vi "Device.Init.vi"(8 "error in (no error)":errorcluster, 11 "OPM.ThorlabsPM400":refnum<class "OPM.ThorlabsPM400.lvclass">) -> (0 "error out":errorcluster, 2 "Result":bool, 3 "OPM.ThorlabsPM400 out":refnum<class "OPM.ThorlabsPM400.lvclass">)   [LabVIEW 2017, in "OPM.ThorlabsPM400.lvclass"]
doc: "---------------------------------------------------------------\nJKI State Machine Objects™\nhttp://jki.net/state-machine-objects/\nCopyright (C) 2005-2015, JKI <info@jki.net>\nALL RIGHTS RESERVEDJKI State Machine Objects (SMO) 1.0.0.5\nJKI - JKI\nCopyright (c) 2016, JKI"
uses:
  OPM.ThorlabsPM400.lvclass
  D:/upwork/Laser Measurement Tool/Laser/project/Subsystems/OPM/OPM.lvclass
  Typedefs/Resource--Cluster.ctl
  OPM/OPM.lvclass
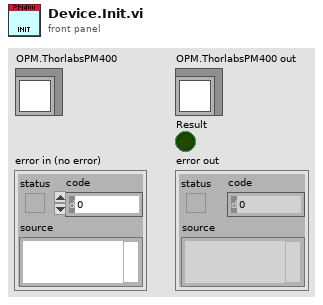
[diagram p1: front panel]
types:
  T1 = typedef "OPM.ThorlabsPM400.lvclass/Resource--Cluster.ctl" = cluster{"Instrument handle":refnum<visa-resource-name>}
  T2 = typedef "OPM.lvclass/Configuration--Cluster.ctl" = cluster{"VISA Resource":string}
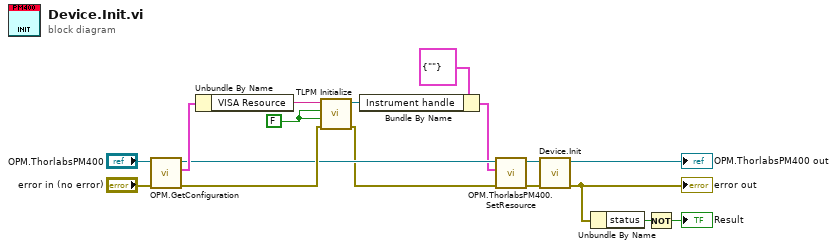
[diagram p0: block diagram]
diagram:
  w12 = FALSE ("ID Query (Do Query)")
  n1 = call "OPM.GetConfiguration.vi"("error in (no error)"="error in (no error)", "PM"="OPM.ThorlabsPM400") -> ("error out"=w11:errorcluster, "Configuration"=w14:T2, "PM out"=w8:refnum<class "OPM.ThorlabsPM400.lvclass">)  [unwired: 7 in]
  n2 = Unbundle By Name(w14) -> ("VISA Resource"=w13:string)
  n3 = call <instrlib>:"TLPM Initialize.vi"("error in (no error)"=w11, "Reset Device (Reset Device)"=w12, "ID Query (Do Query)"=w12, "resource name"=w13) -> ("error out"=w6:errorcluster, "instrument handle out"=w9:refnum<visa-resource-name>)  [unwired: 6 in]
  n4 = Bundle By Name(cluster=T1 {"Instrument handle"=""} ("Resource"), "Instrument handle"=w9) -> (w7:T1)
  n5 = call "OPM.ThorlabsPM400.SetResource.vi"("error in (no error)"=w6, "Resource"=w7, "OPM.ThorlabsPM400 in"=w8) -> ("error out"=w4:errorcluster, "OPM.ThorlabsPM400 out"=w5:refnum<class "OPM.ThorlabsPM400.lvclass">)  [unwired: 7 in]
  n6 = call-parent "Device.Init.vi"("error in (no error)"=w4, "Device in"=w5) -> ("error out"=w2:errorcluster, "Device out"=→"OPM.ThorlabsPM400 out":refnum<class "OPM.ThorlabsPM400.lvclass">)  [unwired: 7 in, 1 out]
  "error out" <- w2
  n7 = Unbundle By Name(w2) -> ("status"=w3:bool)
  n8 = Not(x=w3) -> (.not. x?=→"Result":bool)
